vi "CONTROLES_INTERPRETAR.vi"(6 "Variant":variant, 8 "error in":errorcluster, 9 "name":string, 10 "RD/WR":enum16{"WR", "RD"}(ring)=enum."RD", 11 "Controls[]":refnum<vi>[](array[refnum])) -> (0 "error out":errorcluster, 2 "Value out":variant, 3 "Data":string)   [LabVIEW 2019]
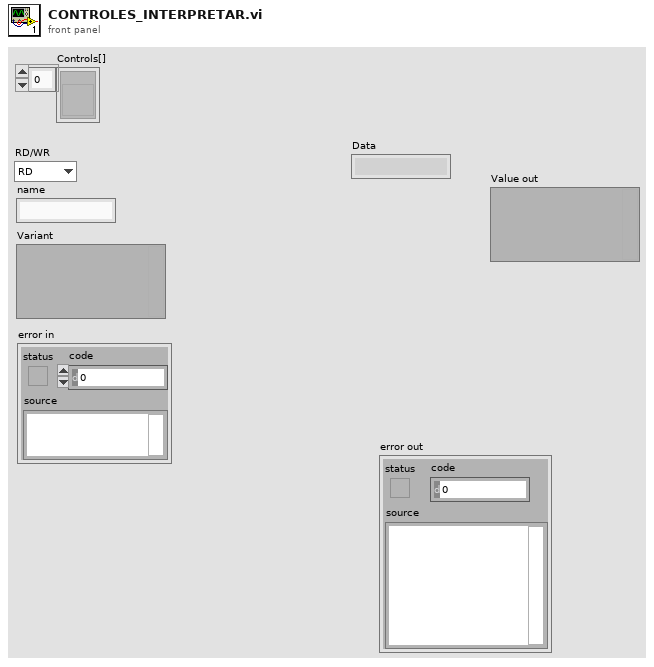
[diagram p1: front panel]
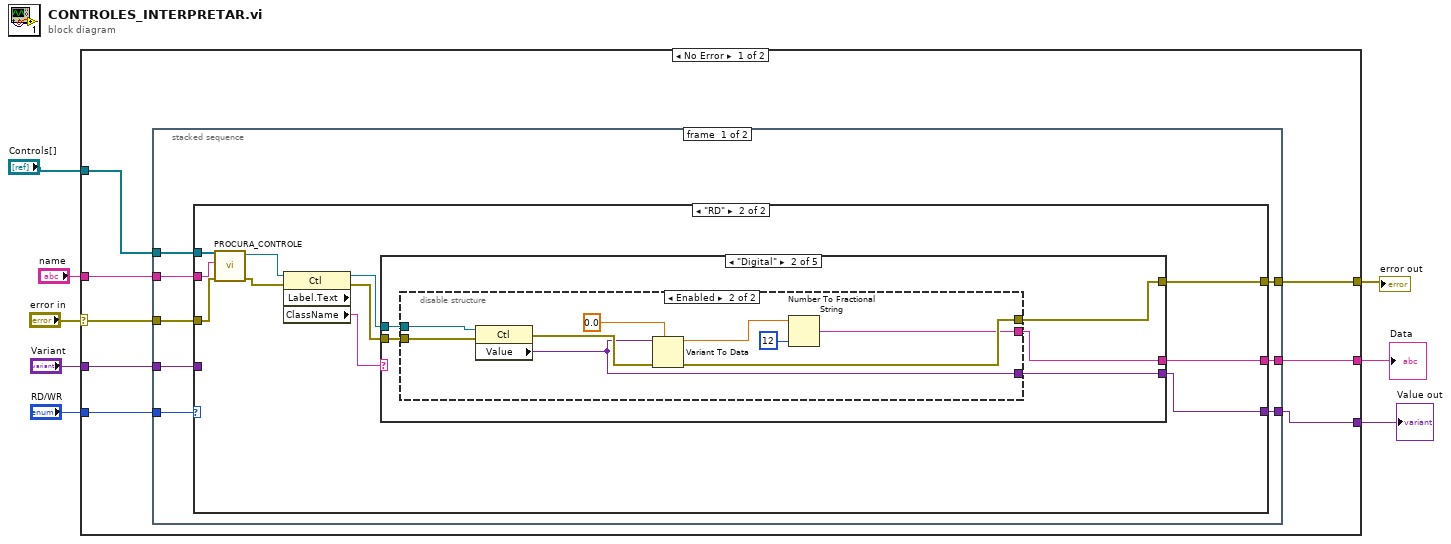
[diagram p0: block diagram]
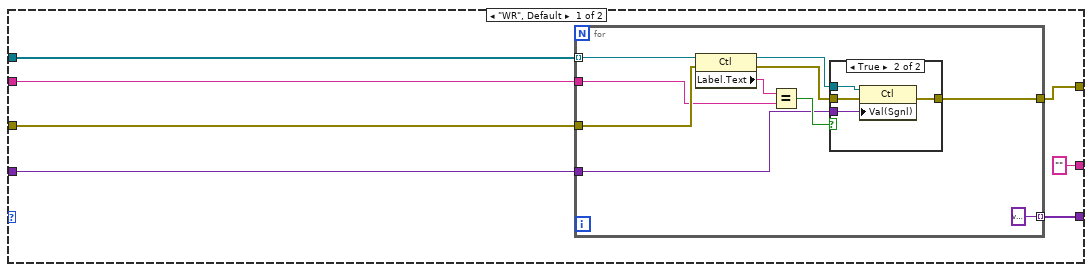
[diagram p2: hidden frame]
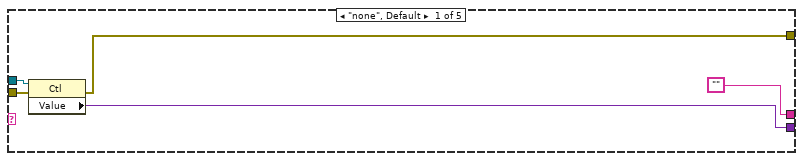
[diagram p4: hidden frame]
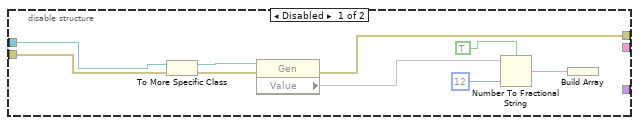
[diagram p5: hidden frame]
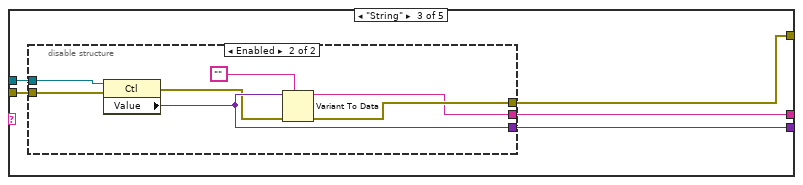
[diagram p6: hidden frame]
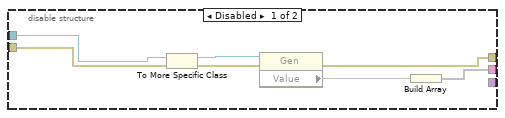
[diagram p7: hidden frame]
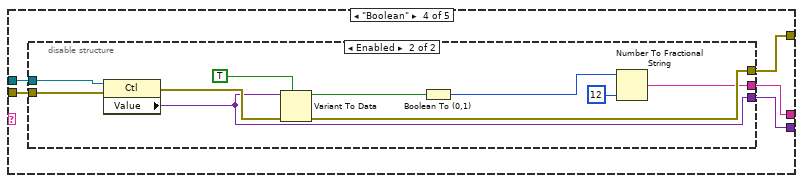
[diagram p8: hidden frame]
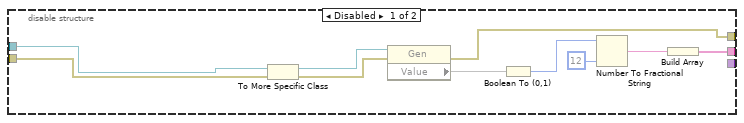
[diagram p9: hidden frame]
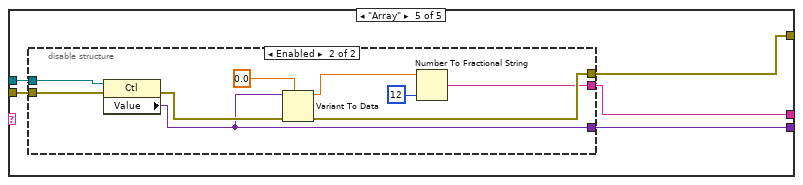
[diagram p10: hidden frame]
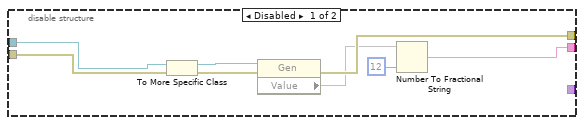
[diagram p11: hidden frame]
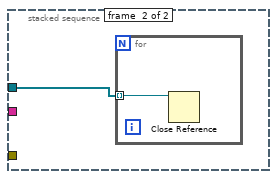
[diagram p12: hidden frame]
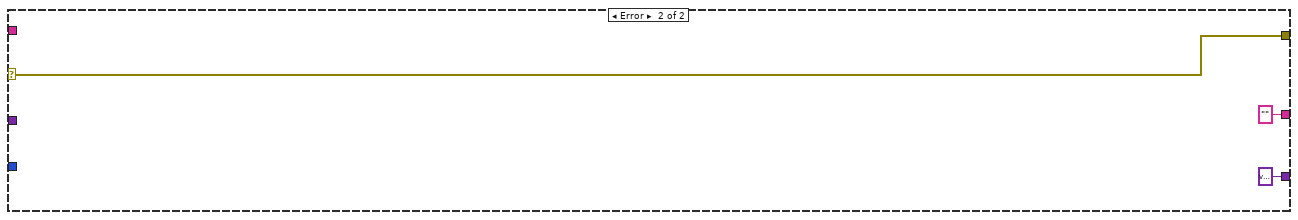
[diagram p13: hidden frame]
diagram:
  n1 = case shown="No Error" "error in" {
    selector: "error in" -> [w16 w163]
    tunnel: [w11 w163] -> w3
    tunnel: "RD/WR" -> [w15 _]
    tunnel: "name" -> [w14 _]
    tunnel: "Variant" -> [w13 _]
    tunnel: "Controls[]" -> [w12 _]
    tunnel: [w10 "" ("Class Name")] -> w2
    tunnel: [w9 variant ("Value")] -> w1
    frame No Error {
      n2 = stacked-sequence {
        tunnel: w16 -> [w24 _]
        tunnel: w15 -> [w23 _]
        tunnel: w14 -> [w22 _]
        tunnel: w13 -> [w21 _]
        tunnel: w12 -> [w20 w159]
        tunnel: [w19 _] -> w11
        tunnel: [w18 _] -> w10
        tunnel: [w17 _] -> w9
        frame #0 {
          n3 = case shown="\"RD\"" w23 {
            tunnel: w20 -> [w31 w55]
            tunnel: w24 -> [w30 w53]
            tunnel: [w29 w56] -> w19
            tunnel: w21 -> [w28 _]
            tunnel: w22 -> [w27 w54]
            tunnel: [w26 w48] -> w17
            tunnel: ["" ("Class Name") w47] -> w18
            frame "WR", Default {
              n4 = for {
                tunnel: w31 -> [w41] mode=indexing
                tunnel: w30 -> [w40]
                tunnel: [w33] -> w29
                tunnel: w28 -> [w35]
                tunnel: w27 -> [w34]
                tunnel: [variant ("Value")] -> w26 mode=indexing
                n5 = property class="Ctl"(reference=w41, error in=w40) -> (reference out=w39:refnum<vi>, error out=w38:errorcluster, "Label.Text"=w37:string)
                n6 = Equal?(x=w37, y=w34) -> (x = y?=w36:bool)
                n7 = case shown="True" w36 {
                  tunnel: w39 -> [_ w46]
                  tunnel: w38 -> [w42 w44]
                  tunnel: [w42 w43] -> w33
                  tunnel: w35 -> [_ w45]
                  frame False {
                  }
                  frame True {
                    n8 = property class="Ctl"(reference=w46, error in=w44, "Val(Sgnl)"=w45) -> (error out=w43:errorcluster)  [unwired: 1 out]
                  }
                }
              }
            }
            frame "RD" {
              n9 = call "PROCURA_CONTROLE.vi"("error in"=w53, "name"=w54, "Controls in"=w55) -> ("error out"=w52:errorcluster, "element"=w49:refnum<vi>)  [unwired: 7 in]
              n10 = property class="Ctl" props=["Label", "Text", "ClassName"](reference=w49, error in=w52) -> (reference out=w51:refnum<vi>, error out=w50:errorcluster, "ClassName"=w57:string)  [unwired: 1 out]
              n11 = case shown="\"Digital\"" w57 {
                tunnel: [w60 w67 w91 w112 w139] -> w56
                tunnel: w51 -> [w62 w66 w90 w110 w138]
                tunnel: w50 -> [w61 w65 w89 w111 w137]
                tunnel: [w59 w64 w88 w109 w136] -> w48
                tunnel: ["" w63 w87 w108 w135] -> w47
                frame "none", Default {
                  n12 = property class="Ctl"(reference=w62, error in=w61) -> (error out=w60:errorcluster, "Value"=w59:variant)  [unwired: 1 out]
                }
                frame "Digital" {
                  n13 = disable-structure shown="Enabled" {
                    disable-tunnel: [w75 w80] -> w67
                    disable-tunnel: w66 -> [w74 w83]
                    disable-tunnel: w65 -> [w73 w82]
                    disable-tunnel: [_ w79] -> w64
                    disable-tunnel: [_ w78] -> w63
                    frame Disabled {
                      n14 = To More Specific Class(reference=w74, error in=w73) -> (target class=w68:refnum<vi>, specific class reference=w77:refnum<vi>, error out=w76:errorcluster)
                      n15 = property class="Gen"(reference=w77, error in=w76) -> (error out=w75:errorcluster, "Value"=w72)  [unwired: 1 out]
                      n16 = Number To Fractional String(use system decimal point (T)=TRUE, number=w72, precision (6)=i16 12) -> (F-format string=w70:string)  [unwired: 1 in]
                      n17 = Build Array(w70) -> ()  [unwired: 1 out]
                    }
                    frame Enabled {
                      n18 = property class="Ctl"(reference=w83, error in=w82) -> (error out=w86:errorcluster, "Value"=w79:variant)  [unwired: 1 out]
                      n19 = Variant To Data(error in=w86, type=0.0 ("Numeric"), Variant=w79) -> (data=w84:dbl, error out=w80:errorcluster)
                      n20 = Number To Fractional String(number=w84, precision (6)=i16 12) -> (F-format string=w78:string)  [unwired: 2 in]
                    }
                  }
                }
                frame "String" {
                  n21 = disable-structure shown="Enabled" {
                    disable-tunnel: [w99 w102] -> w91
                    disable-tunnel: w90 -> [w97 w107]
                    disable-tunnel: w89 -> [w95 w106]
                    disable-tunnel: [w94 w101] -> w87
                    disable-tunnel: [_ w104] -> w88
                    frame Disabled {
                      n22 = To More Specific Class(reference=w97, error in=w95) -> (target class=w92:refnum<vi>, specific class reference=w98:refnum<vi>, error out=w96:errorcluster)
                      n23 = property class="Gen"(reference=w98, error in=w96) -> (reference out=w100:refnum<vi>, error out=w99:errorcluster, "Value"=w93)
                      n24 = Build Array(w93) -> (w94:void[])
                    }
                    frame Enabled {
                      n25 = property class="Ctl"(reference=w107, error in=w106) -> (error out=w103:errorcluster, "Value"=w104:variant)  [unwired: 1 out]
                      n26 = Variant To Data(error in=w103, type="" ("Class Name"), Variant=w104) -> (data=w101:string, error out=w102:errorcluster)
                    }
                  }
                }
                frame "Boolean" {
                  n27 = disable-structure shown="Enabled" {
                    disable-tunnel: [w123 w127] -> w112
                    disable-tunnel: w111 -> [w121 w133]
                    disable-tunnel: w110 -> [w120 w134]
                    disable-tunnel: [w117 w125] -> w108
                    disable-tunnel: [_ w126] -> w109
                    frame Disabled {
                      n28 = To More Specific Class(reference=w120, error in=w121) -> (target class=w113:refnum<vi>, specific class reference=w119:refnum<vi>, error out=w122:errorcluster)
                      n29 = property class="Gen"(reference=w119, error in=w122) -> (reference out=w124:refnum<vi>, error out=w123:errorcluster, "Value"=w118)
                      n30 = Boolean To (0,1)(Boolean=w118) -> (0, 1=w115:i16)
                      n31 = Number To Fractional String(number=w115, precision (6)=i16 12) -> (F-format string=w116:string)  [unwired: 2 in]
                      n32 = Build Array(w116) -> (w117:string[])
                    }
                    frame Enabled {
                      n33 = property class="Ctl"(reference=w134, error in=w133) -> (error out=w132:errorcluster, "Value"=w126:variant)  [unwired: 1 out]
                      n34 = Variant To Data(error in=w132, type=TRUE, Variant=w126) -> (data=w128:bool, error out=w127:errorcluster)
                      n35 = Boolean To (0,1)(Boolean=w128) -> (0, 1=w130:i16)
                      n36 = Number To Fractional String(number=w130, precision (6)=i16 12) -> (F-format string=w125:string)  [unwired: 2 in]
                    }
                  }
                }
                frame "Array" {
                  n37 = disable-structure shown="Enabled" {
                    disable-tunnel: [w148 w155] -> w139
                    disable-tunnel: w138 -> [w145 w157]
                    disable-tunnel: w137 -> [w144 w156]
                    disable-tunnel: [w141 w153] -> w135
                    disable-tunnel: [_ w152] -> w136
                    frame Disabled {
                      n38 = To More Specific Class(reference=w145, error in=w144) -> (target class=w140:refnum<vi>, specific class reference=w146:refnum<vi>, error out=w147:errorcluster)
                      n39 = property class="Gen"(reference=w146, error in=w147) -> (reference out=w149:refnum<vi>, error out=w148:errorcluster, "Value"=w142)
                      n40 = Number To Fractional String(number=w142, precision (6)=i16 12) -> (F-format string=w141:string)  [unwired: 2 in]
                    }
                    frame Enabled {
                      n41 = property class="Ctl"(reference=w157, error in=w156) -> (error out=w158:errorcluster, "Value"=w152:variant)  [unwired: 1 out]
                      n42 = Variant To Data(error in=w158, type=0.0, Variant=w152) -> (data=w150:dbl, error out=w155:errorcluster)
                      n43 = Number To Fractional String(number=w150, precision (6)=i16 12) -> (F-format string=w153:string)  [unwired: 2 in]
                    }
                  }
                }
              }
            }
          }
        }
        frame #1 {
          n44 = for {
            tunnel: w159 -> [w160] mode=indexing
            n45 = Close Reference(reference=w160) -> ()  [unwired: 1 in, 1 out]
          }
        }
      }
    }
    frame Error {
    }
  }
  "error out" <- w3
  "Data" <- w2
  "Value out" <- w1
